vi "ramps convert.vi"(4 "End time 10us":i32, 6 "Ramp3 time 10us":i32, 7 "Amp":dbl, 9 "Ramp2 time 10us":i32, 10 "Ramp1 time 10us":i32, 11 "Delay time 10us":i32) -> (3 "Ramps cluster":T1)   [LabVIEW 2024]
uses:
  cRIO related/Ramps.ctl
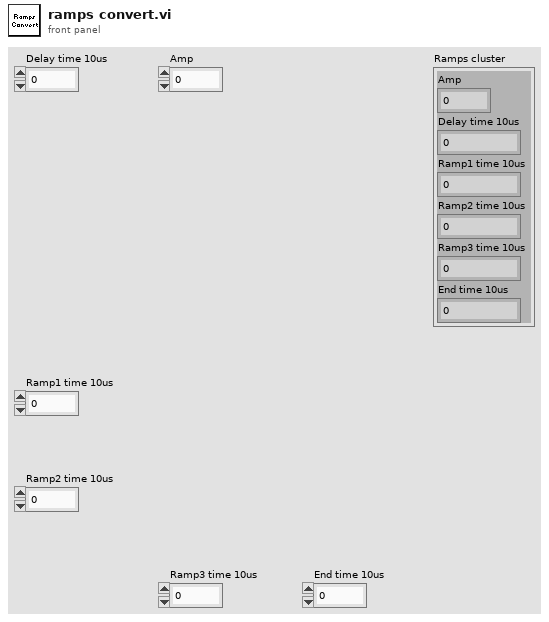
[diagram p1: front panel]
types:
  T1 = typedef "Ramps.ctl" = cluster{"Amp":fxp<+/-,20,5>, "Delay time 10us":i32, "Ramp1 time 10us":i32, "Ramp2 time 10us":i32, "Ramp3 time 10us":i32, "End time 10us":i32}
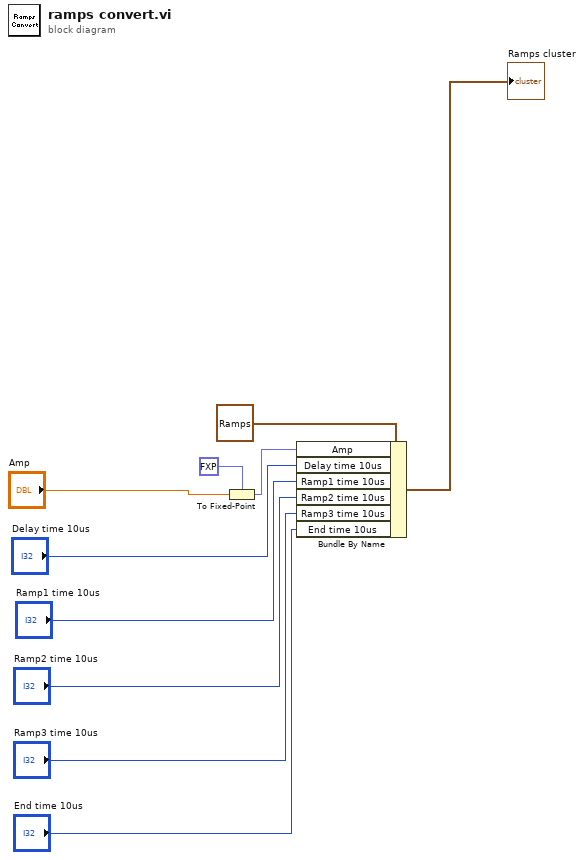
[diagram p0: block diagram]
diagram:
  n1 = To Fixed-Point(fixed-point type=fxp<+/-,20,5> 0.0 ("Amp"), number="Amp") -> (fixed-point=w4:fxp<+/-,20,5>)
  n2 = Bundle By Name(cluster=T1 {"Amp"=1.5, "Delay time 10us"=1000, "Ramp1 time 10us"=1000, "Ramp2 time 10us"=2000, "Ramp3 time 10us"=1000, "End time 10us"=0} ("Ramps cluster"), "Amp"=w4, "Delay time 10us"="Delay time 10us", "Ramp1 time 10us"="Ramp1 time 10us", "Ramp2 time 10us"="Ramp2 time 10us", "Ramp3 time 10us"="Ramp3 time 10us", "End time 10us"="End time 10us") -> (→"Ramps cluster":T1)
